vi "Wait for User to Soft Trigger.vi"(9 "occurrence":refnum<k4>, 10 "Soft Trigger In":bool) -> (2 "Soft Trigger Out":bool)   [LabVIEW 2017, in "DTACQ - Network Enabled Device Driver.lvlib"]
doc: "Waits for the user to click the button, if soft trigger is enabled."
uses:
  DTACQ - Network Enabled Device Driver.lvlib
panel:
  in  "Fire Button":bool
  # "Fire Soft Trigger"
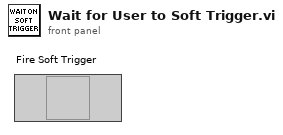
[diagram p1: front panel]
types:
  T1 = enum32{"Invalid", "Standard", "Closed", "Hidden", "Minimized", "Maximized"}
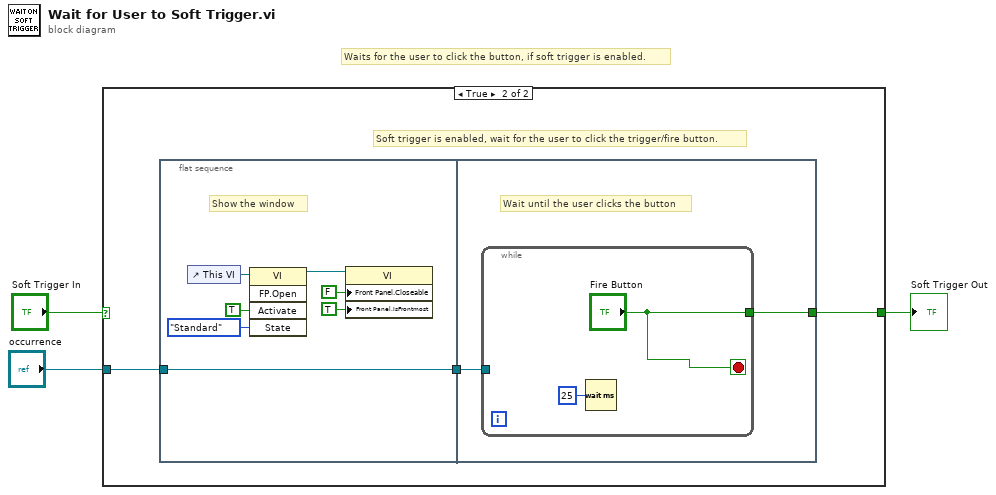
[diagram p0: block diagram]
diagram:
  # "Waits for the user to click the button, if soft trigger is enabled."
  n1 = case shown="True" "Soft Trigger In" {
    selector: "Soft Trigger In" -> [w4 _]
    tunnel: [w4 w7] -> w3
    tunnel: "occurrence" -> [_ w6]
    frame False {
      # "Soft trigger is disabled, proceed immediately"
    }
    frame True {
      # "Soft trigger is enabled, wait for the user to click the trigger/fire button."
      n2 = flat-sequence {
        tunnel: w6 -> [w8]
        tunnel: [w8] -> w5
        tunnel: [w16] -> w7
        tunnel: w5 -> [w15]
        frame #0 {
          # "Show the window"
          n3 = control-ref of="This VI"() -> (w14:refnum<vi>)
          n4 = invoke class="VI" method="FP.Open"(reference=w14, "Activate"=TRUE ("Activate?"), "State"=T1."Standard") -> (reference out=w11:refnum<vi>)  [unwired: 2 in, 4 out]
          n5 = property class="VI"(reference=w11, "Front Panel.Closeable"=FALSE ("Front Panel Window:Closeable"), "Front Panel.IsFrontmost"=TRUE ("Front Panel Window:Is Frontmost")) -> ()  [unwired: 1 in, 2 out]
        }
        frame #1 {
          # "Wait until the user clicks the button"
          n6 = while {
            tunnel: ["Fire Button"] -> w16
            tunnel: w15 -> [_]
            stop <- "Fire Button" stop-if-true
            n7 = Wait (ms)(milliseconds to wait=u32 25) -> ()  [unwired: 1 out]
          }
        }
      }
    }
  }
  "Soft Trigger Out" <- w3
